vi "sub_GSlam_cal-edge.vi"(11 "in":T3) -> (3 "edge out":T2={"e"=[[0.04000000000000001]], "omega"=[[0.04000000000000001]], "d1"=0.0, "d2"=0.0, "yaw1"=0.0, "yaw2"=0.0, "angle1"=0.0, "angle2"=0.0, "id1"=0, "id2"=0})   [LabVIEW 2019]
uses:
  Ctrl/slam_edge.ctl
  <vilib>/Analysis/Matrix/Datatypes/RealMatrix.ctl
  <vilib>/Analysis/coordinate.llb/Euler Rotation Order.ctl
  <vilib>/Analysis/Matrix/Numeric/Conversions/Array To Matrix - RA.vi
  <vilib>/Analysis/Matrix/Numeric/Conversions/Array To Matrix - RA2.vi
  <vilib>/Analysis/Matrix/Numeric/Multiply/Multiply - RM,RM.vi
  <vilib>/Analysis/Matrix/Numeric/Add/Add - RM,RM.vi
  <vilib>/Analysis/baseanly.llb/Real Inverse Matrix.vi
  <vilib>/Analysis/Matrix/NI_Matrix.lvlib
  <vilib>/Analysis/NI_AALPro.lvlib
  <vilib>/Analysis/NI_AALBase.lvlib
panel:
  out "강도 그래프":dbl[][](graph)
  out "sigma":T1
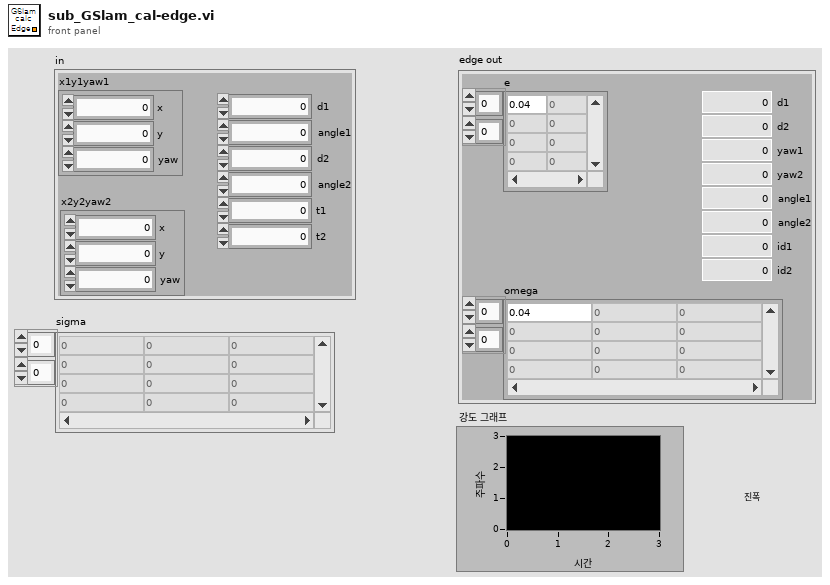
[diagram p1: front panel]
types:
  T1 = typedef "NI_Matrix.lvlib/RealMatrix.ctl" = dbl[][]
  T2 = typedef "slam_edge.ctl" = cluster{"e":T1, "omega":T1, "d1":dbl, "d2":dbl, "yaw1":dbl, "yaw2":dbl, "angle1":dbl, "angle2":dbl, "id1":i32, "id2":i32}
  T3 = cluster{"x1y1yaw1":cluster{"x":dbl, "y":dbl, "yaw":dbl}, "x2y2yaw2":cluster{"x":dbl, "y":dbl, "yaw":dbl}, "d1":dbl, "angle1":dbl, "d2":dbl, "angle2":dbl, "t1":i32, "t2":i32}
  T4 = typedef "NI_AALPro.lvlib/Euler Rotation Order.ctl" = u16
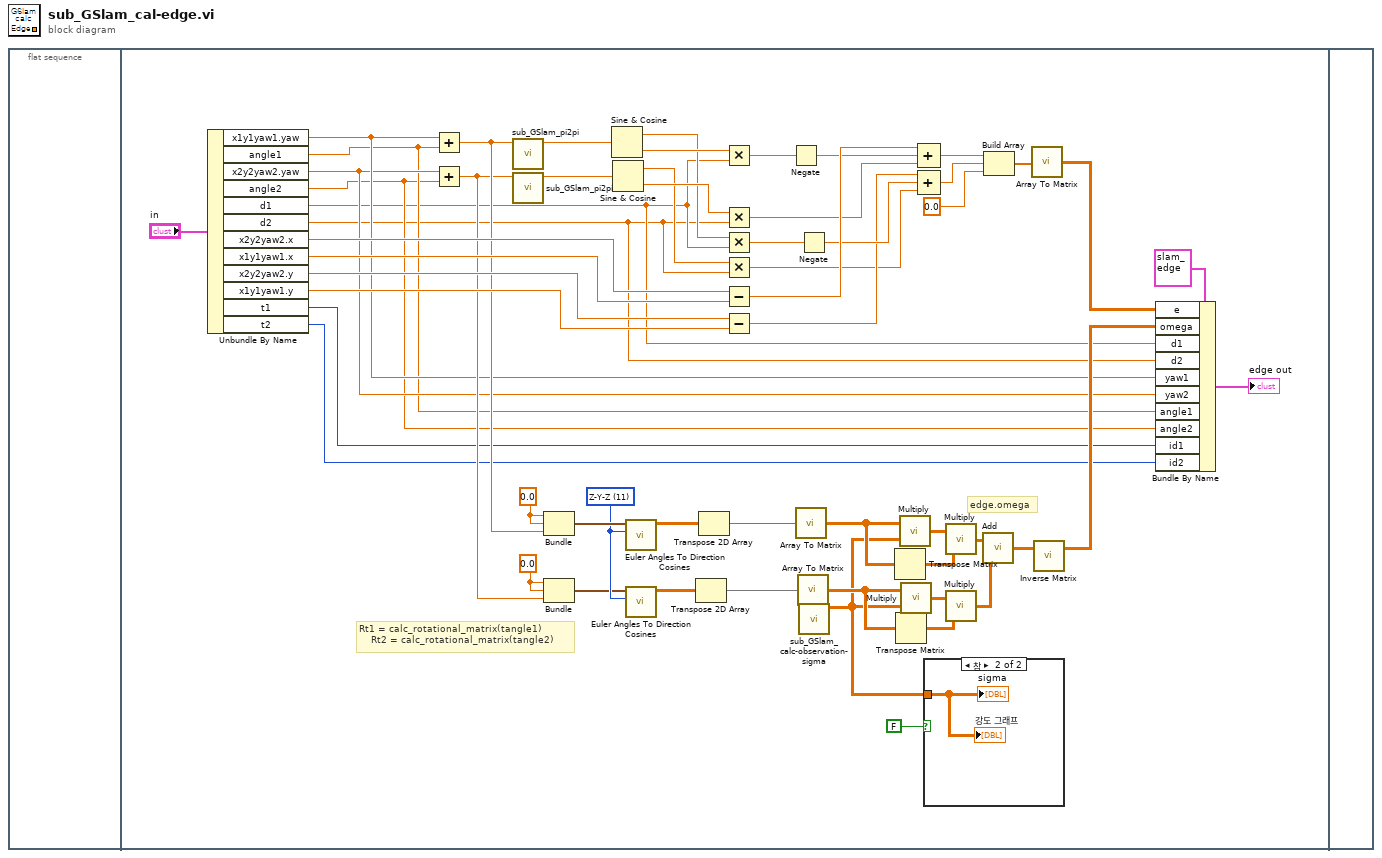
[diagram p0: block diagram]
diagram:
  n1 = flat-sequence {
    frame #0 {
    }
    frame #1 {
      w28 = T4 11 items=["X-Y-Z", "X-Z-Y", "Y-X-Z", "Y-Z-X", "Z-X-Y", "Z-Y-X", "X-Y-X", "X-Z-X", "Y-X-Y", "Y-Z-Y", "Z-X-Z", "Z-Y-Z"] ("rotation order")
      w31 = 0.0 ("원소")
      w33 = 0.0 ("원소")
      # "edge.omega"
      # "Rt1 = calc_rotational_matrix(tangle1)\n    Rt2 = calc_rotational_matrix(tangle2)"
      n2 = Unbundle By Name("in") -> ("x1y1yaw1.yaw"=w14:dbl, "angle1"=w12:dbl, "x2y2yaw2.yaw"=w13:dbl, "angle2"=w11:dbl, "d1"=w10:dbl, "d2"=w9:dbl, "x2y2yaw2.x"=w50:dbl, "x1y1yaw1.x"=w49:dbl, "x2y2yaw2.y"=w45:dbl, "x1y1yaw1.y"=w44:dbl, "t1"=w8:i32, "t2"=w7:i32)
      n3 = Add(x=w14, y=w12) -> (x+y=w32:dbl)
      n4 = Add(x=w13, y=w11) -> (x+y=w30:dbl)
      n5 = call "sub_GSlam_pi2pi.vi"("angle"=w32) -> ("result"=w56:dbl)  [unwired: 10 in]
      n6 = call "sub_GSlam_pi2pi.vi"("angle"=w30) -> ("result"=w55:dbl)  [unwired: 10 in]
      n7 = Bundle("원소"=w33, "원소"=w33, w32) -> (w29:cluster{"원소":dbl, "원소":dbl, dbl})  [unwired: 1 in]
      n8 = Bundle("원소"=w31, "원소"=w31, w30) -> (w27:cluster{"원소":dbl, "원소":dbl, dbl})  [unwired: 1 in]
      n9 = Sine & Cosine(0:w56) -> (1:w52:dbl, 2:w54:dbl)
      n10 = Sine & Cosine(0:w55) -> (1:w51:dbl, 2:w53:dbl)
      n11 = call <vilib>:"Euler Angles To Direction Cosines.vi"("rotation order"=w28, "Euler Angles"=w29) -> ("Direction Cosines"=w26:dbl[][])  [unwired: 8 in, 1 out]
      n12 = call <vilib>:"Euler Angles To Direction Cosines.vi"("rotation order"=w28, "Euler Angles"=w27) -> ("Direction Cosines"=w20:dbl[][])  [unwired: 8 in, 1 out]
      n13 = Transpose 2D Array(2D array=w20) -> (transposed array=w2:dbl[][])
      n14 = Transpose 2D Array(2D array=w26) -> (transposed array=w3:dbl[][])
      n15 = Multiply ("tmp1")(x=w54, y=w10) -> (x*y=w47:dbl)
      n16 = Multiply ("tmp2")(x=w53, y=w9) -> (x*y=w43:dbl)
      n17 = Multiply ("tmp3")(x=w52, y=w10) -> (x*y=w40:dbl)
      n18 = Multiply ("tmp4")(x=w51, y=w9) -> (x*y=w39:dbl)
      n19 = Subtract(x=w50, y=w49) -> (x-y=w48:dbl)
      n20 = Subtract(x=w45, y=w44) -> (x-y=w41:dbl)
      n21 = Negate(x=w47) -> (-x=w46:dbl)
      n22 = call-poly <vilib>:"Array To Matrix.vi"("Real 2D Array"=w3) -> ("Real Matrix"=w23:T1)
      n23 = call-poly <vilib>:"Array To Matrix.vi"("Real 2D Array"=w2) -> ("Real Matrix"=w19:T1)
      n24 = Negate(x=w40) -> (-x=w42:dbl)
      n25 = call "sub_GSlam_calc-observation-sigma.vi"() -> ("sigma"=w4:T1)  [unwired: 11 in]
      n26 = Transpose Matrix(1:w23) -> (0:w24:T1)
      n27 = Transpose Matrix(1:w19) -> (0:w22:T1)
      n28 = call-poly <vilib>:"Multiply.vi"("Real Matrix B"=w4, "Real Matrix A"=w23) -> ("A * B"=w25:T1)
      n29 = call-poly <vilib>:"Multiply.vi"("Real Matrix B"=w4, "Real Matrix A"=w19) -> ("A * B"=w21:T1)
      n30 = Compound Arithmetic op=ADD(w48, w46, w43) -> (w38:dbl)
      n31 = Compound Arithmetic op=ADD(w41, w42, w39) -> (w37:dbl)
      n32 = case shown="참" FALSE {
        tunnel: w4 -> [_ w58]
        frame False {
        }
        frame True {
          "sigma" <- w58
          "강도 그래프" <- w58
        }
      }
      n33 = call-poly <vilib>:"Multiply.vi"("Real Matrix B"=w24, "Real Matrix A"=w25) -> ("A * B"=w18:T1)
      n34 = call-poly <vilib>:"Multiply.vi"("Real Matrix B"=w22, "Real Matrix A"=w21) -> ("A * B"=w17:T1)
      n35 = call-poly <vilib>:"Add.vi"("Real Matrix B"=w17, "Real Matrix A"=w18) -> ("A + B"=w16:T1)
      n36 = Build Array(w38, w37, 0.0 ("원소")) -> (w35:dbl[])
      n37 = call-poly <vilib>:"Array To Matrix.vi"("Real 1D Array"=w35) -> ("Real Matrix (Column Vector)"=w34:T1)
      n38 = call-poly <vilib>:"Inverse Matrix.vi"("Input Matrix"=w16) -> ("Inverse Matrix"=w15:T1)  [unwired: 1 in, 1 out]
      n39 = Bundle By Name(cluster=T2 {"e"=[[0.0], [0.0], [0.0]], "omega"=[[0.0, 0.0, 0.0], [0.0, 0.0, 0.0], [-0.0, -0.0, 0.0]], "d1"=0.0, "d2"=0.0, "yaw1"=0.0, "yaw2"=0.0, "angle1"=0.0, "angle2"=0.0, "id1"=0, "id2"=0} ("pf-val out"), "e"=w34, "omega"=w15, "d1"=w10, "d2"=w9, "yaw1"=w14, "yaw2"=w13, "angle1"=w12, "angle2"=w11, "id1"=w8, "id2"=w7) -> (→"edge out":T2)
    }
    frame #2 {
    }
  }
